vi "Z900_navX_Open_I2C.vi"(8 "error in (no error)":errorcluster, 10 "I2C Bus":T1=enum."Invalid", 11 "Update Rate (4Hz-60Hz)":u8=50 min=4 max=60 step=1) -> (0 "error out":errorcluster, 3 "navX Device":T2={"Interface"={"Protocol"=enum."SERIAL", "Update Rate (4Hz-60Hz)"=4, "navX Open TypeDef"=variant}, "Notify Packet"=refnum, "Loop VI Refnum"=refnum, "Ready to Close Occurrence Refnum"=refnum} {"Interface"."Update Rate (4Hz-60Hz)" min=4 max=60 step=1})   [LabVIEW 2015, in "navX Library v2.lvlib"]
doc: "This VI opens the navX over I2C. You must open a reference before using any other VIs on this palette. After you open a reference to the navX, you can use the other navX VIs to access and monitor the navX device."
uses:
  navX Library v2.lvlib
  TypeDefs/Z900_navX_DeviceTypeDef.ctl
  TypeDefs/Z900_navX_ProtocolTypeDef.ctl
  TypeDefs/Z900_navX_NotifyPacketTypeDef.ctl
  TypeDefs/Z900_navX_ActionTypeDef.ctl
  <vilib>/Rock Robotics/SystemInterfaces/i2clib/i2c_bus.ctl
  TypeDefs/navX Open TypeDefs/Z900_navX_OpenTypeDef_I2C.ctl
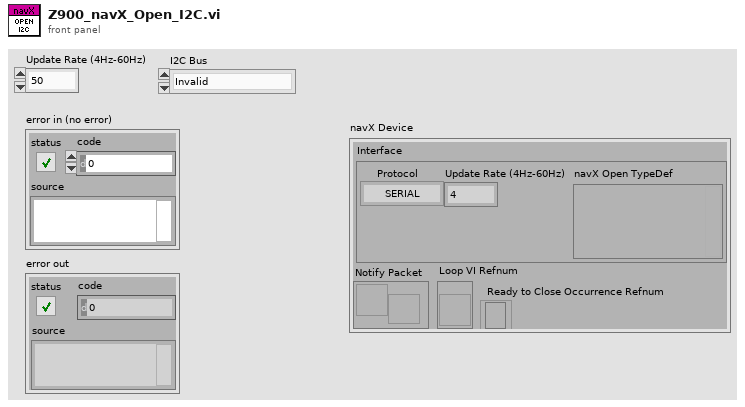
[diagram p1: front panel]
types:
  T1 = typedef "i2c_bus.ctl" = enum16{"I2C On-Board", "I2C MXP", "Invalid"}
  T2 = typedef "navX Library v2.lvlib/Z900_navX_DeviceTypeDef.ctl" = cluster{"Interface":cluster{"Protocol":T3, "Update Rate (4Hz-60Hz)":u8, "navX Open TypeDef":variant}, "Notify Packet":refnum<notifier>, "Loop VI Refnum":refnum<vi>, "Ready to Close Occurrence Refnum":refnum<k4>}
  T3 = typedef "navX Library v2.lvlib/Z900_navX_ProtocolTypeDef.ctl" = enum16{"SERIAL", "I2C", "SPI"}
  T4 = typedef "navX Library v2.lvlib/Z900_navX_OpenTypeDef_I2C.ctl" = cluster{"I2C Bus":T1}
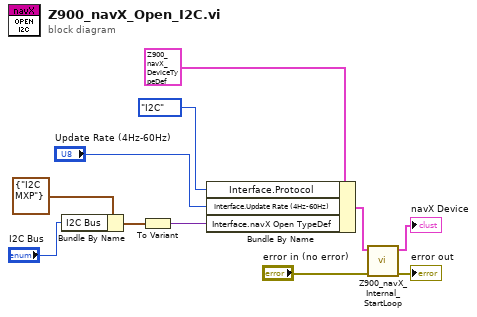
[diagram p0: block diagram]
diagram:
  n1 = Bundle By Name(cluster=T4 {"I2C Bus"=enum."I2C MXP"} ("navX I2C Open"), "I2C Bus"="I2C Bus") -> (w2:T4)
  n2 = To Variant(anything=w2) -> (Variant=w1:variant)
  n3 = Bundle By Name(cluster=T2 {"Interface"={"Protocol"=enum."SERIAL", "Update Rate (4Hz-60Hz)"=0, "navX Open TypeDef"=variant}, "Notify Packet"=refnum, "Loop VI Refnum"=refnum, "Ready to Close Occurrence Refnum"=refnum} ("navX Device"), "Interface.Protocol"=Z900_navX_ProtocolTypeDef."I2C", "Interface.Update Rate (4Hz-60Hz)"="Update Rate (4Hz-60Hz)", "Interface.navX Open TypeDef"=w1) -> (w8:T2)
  n4 = call "Z900_navX_Internal_StartLoop.vi"("error in (no error)"="error in (no error)", "navX Device"=w8) -> ("error out"=→"error out":errorcluster, "navX Device"=→"navX Device":T2)  [unwired: 8 in]
